vi "auto_id_subv.vi"(8 "error in":errorcluster, 9 "Amplitude":dbl=0.15 format="%#_13g", 10 "Bode amplitude 2":refnum<vi>, 11 "Swept-Sines-Control-Settings":cluster{"u-max":sgl, "offset":sgl, "Ki":sgl}) -> (0 "error out":errorcluster, 1 "Is-Totally-Stable":bool, 2 "Dinv-den":dbl[](array[numeric]) format="%#_10g", 3 "Dinv-num":dbl[](array[numeric]) format="%#_10g", 4 "fit_sos_result":T4)   [LabVIEW 2017]
uses:
  controls/SS_SweptSines.ctl
  controls/SS_sin_params.ctl
  controls/SS_input_data_json.ctl
  controls/fit_sos_results.ctl
  controls/SS_figures.ctl
  controls/bode_figure.ctl
  controls/SOS_frf_data.ctl
  controls/logging_selection.ctl
  <vilib>/Utility/error.llb/DialogType.ctl
  <vilib>/FPGAPlugInAG/cRIO-9082/niLvFpga_Open_cRIO-9082.vi
  <vilib>/rvi/interface/common/dynamic/niFpgaDynamicAddResources.vi
  <vilib>/FPGAPlugInAG/Dynamic/niLvFpga_Reset_Dynamic.vi
  <vilib>/rvi/interface/common/niFpgaWaitOnOcc.vi
  <vilib>/Utility/error.llb/Error Cluster From Error Code.vi
  <vilib>/rvi/errors/niLvFpgaAdjustHostInterfaceError.vi
  <vilib>/FPGAPlugInAG/Dynamic/niLvFpga_Run_Dynamic.vi
  <vilib>/FPGAPlugInAG/Dynamic/niLvFpga_Close_Dynamic.vi
  <vilib>/rvi/interface/nirviOpenFPGA/nirviOpenFPGA.xnode
  FPGA Bitfiles/SS_fpga_swept_sines.lvbitx
  <vilib>/rvi/interface/nirviMethod/nirviMethod.xnode
  <vilib>/rvi/interface/nirviReadWriteControl/nirviReadWriteControl.xnode
  <vilib>/rvi/interface/nirviCloseFPGA/nirviCloseFPGA.xnode
  NiFpgaLv.dll
  labview/utils_lib/utils.lvlib
  <vilib>/rvi/interface/Simulation/niFpgaSimulationCallBeginRW.vi
  <vilib>/FPGAPlugInAG/Dynamic/niLvFpga_ConfigureFifo_Dynamic.vi
  <vilib>/rvi/errors/niLvFpgaMergeErrorWithErrorCode.vi
panel:
  out "NaN/Path/Refnum?":bool
  in  "theta0":dbl[](array[numeric])=[0.6786, -1.9959, 0.99891, -1.996142, 0.9989]
  out "Freqs Done":i32(slide) scale=0.0..50.0
  out "SweptSines (out)":T1={"Log-Channel_select"=[FALSE, FALSE, FALSE, FALSE, FALSE, FALSE], "JSON Header"="", "SS-Params-Array"=[], "input_frequency_definitions"={"Amp"=0.0, "Ts"=0.0, "num_periodsMT"=[], "freqs_Hz"=[], "numAve_s"=[], "Nsamp_total"=[], "Nsettle_s"=[], "Ncollect_s"=[]}, "DAC-ADC primary 2"=0, "Channel-Names"=[], "num_chan"=0, "num-freqs"=0, "Input File (json)"=path "Z:/mpc-journal/sysID/FRF_data/x-axis_sines_info.json"} {"DAC-ADC primary 2" items=["DAC0/ADC0", "DAC1/ADC1", "DAC2/ADC2", "DAC3/ADC3", ""]}
  in  "Input File (json)":path=path "Z:/afm-cs/sysID/z-axis_sines_info_quick_firstRes.json"
  out "theta-fit":dbl[](array[numeric])
  out "Bode amplitude":cluster{"W":dbl[], "Magnitude":dbl[]}[](graph) caption="Magnitude Graph"
  in  "SweptSines (in)":T1={"Log-Channel_select"=[FALSE, FALSE, FALSE, FALSE, FALSE, FALSE], "JSON Header"="", "SS-Params-Array"=[], "input_frequency_definitions"={"Amp"=0.0, "Ts"=0.0, "num_periodsMT"=[], "freqs_Hz"=[], "numAve_s"=[], "Nsamp_total"=[], "Nsettle_s"=[], "Ncollect_s"=[]}, "DAC-ADC primary 2"=0, "Channel-Names"=[], "num_chan"=0, "num-freqs"=0, "Input File (json)"=path "Z:/afm-cs/sysID/x-axis_sines_info_intsamps_quick.json"} {"DAC-ADC primary 2" items=["DAC0/ADC0", "DAC1/ADC1", "DAC2/ADC2", "DAC3/ADC3", ""]}
  out "TsTicks":u32
  out "freq_adjusted":dbl
  in  "ABORT":bool
  out "boolean  indicators":T5
  out "number_of_freqs":i32
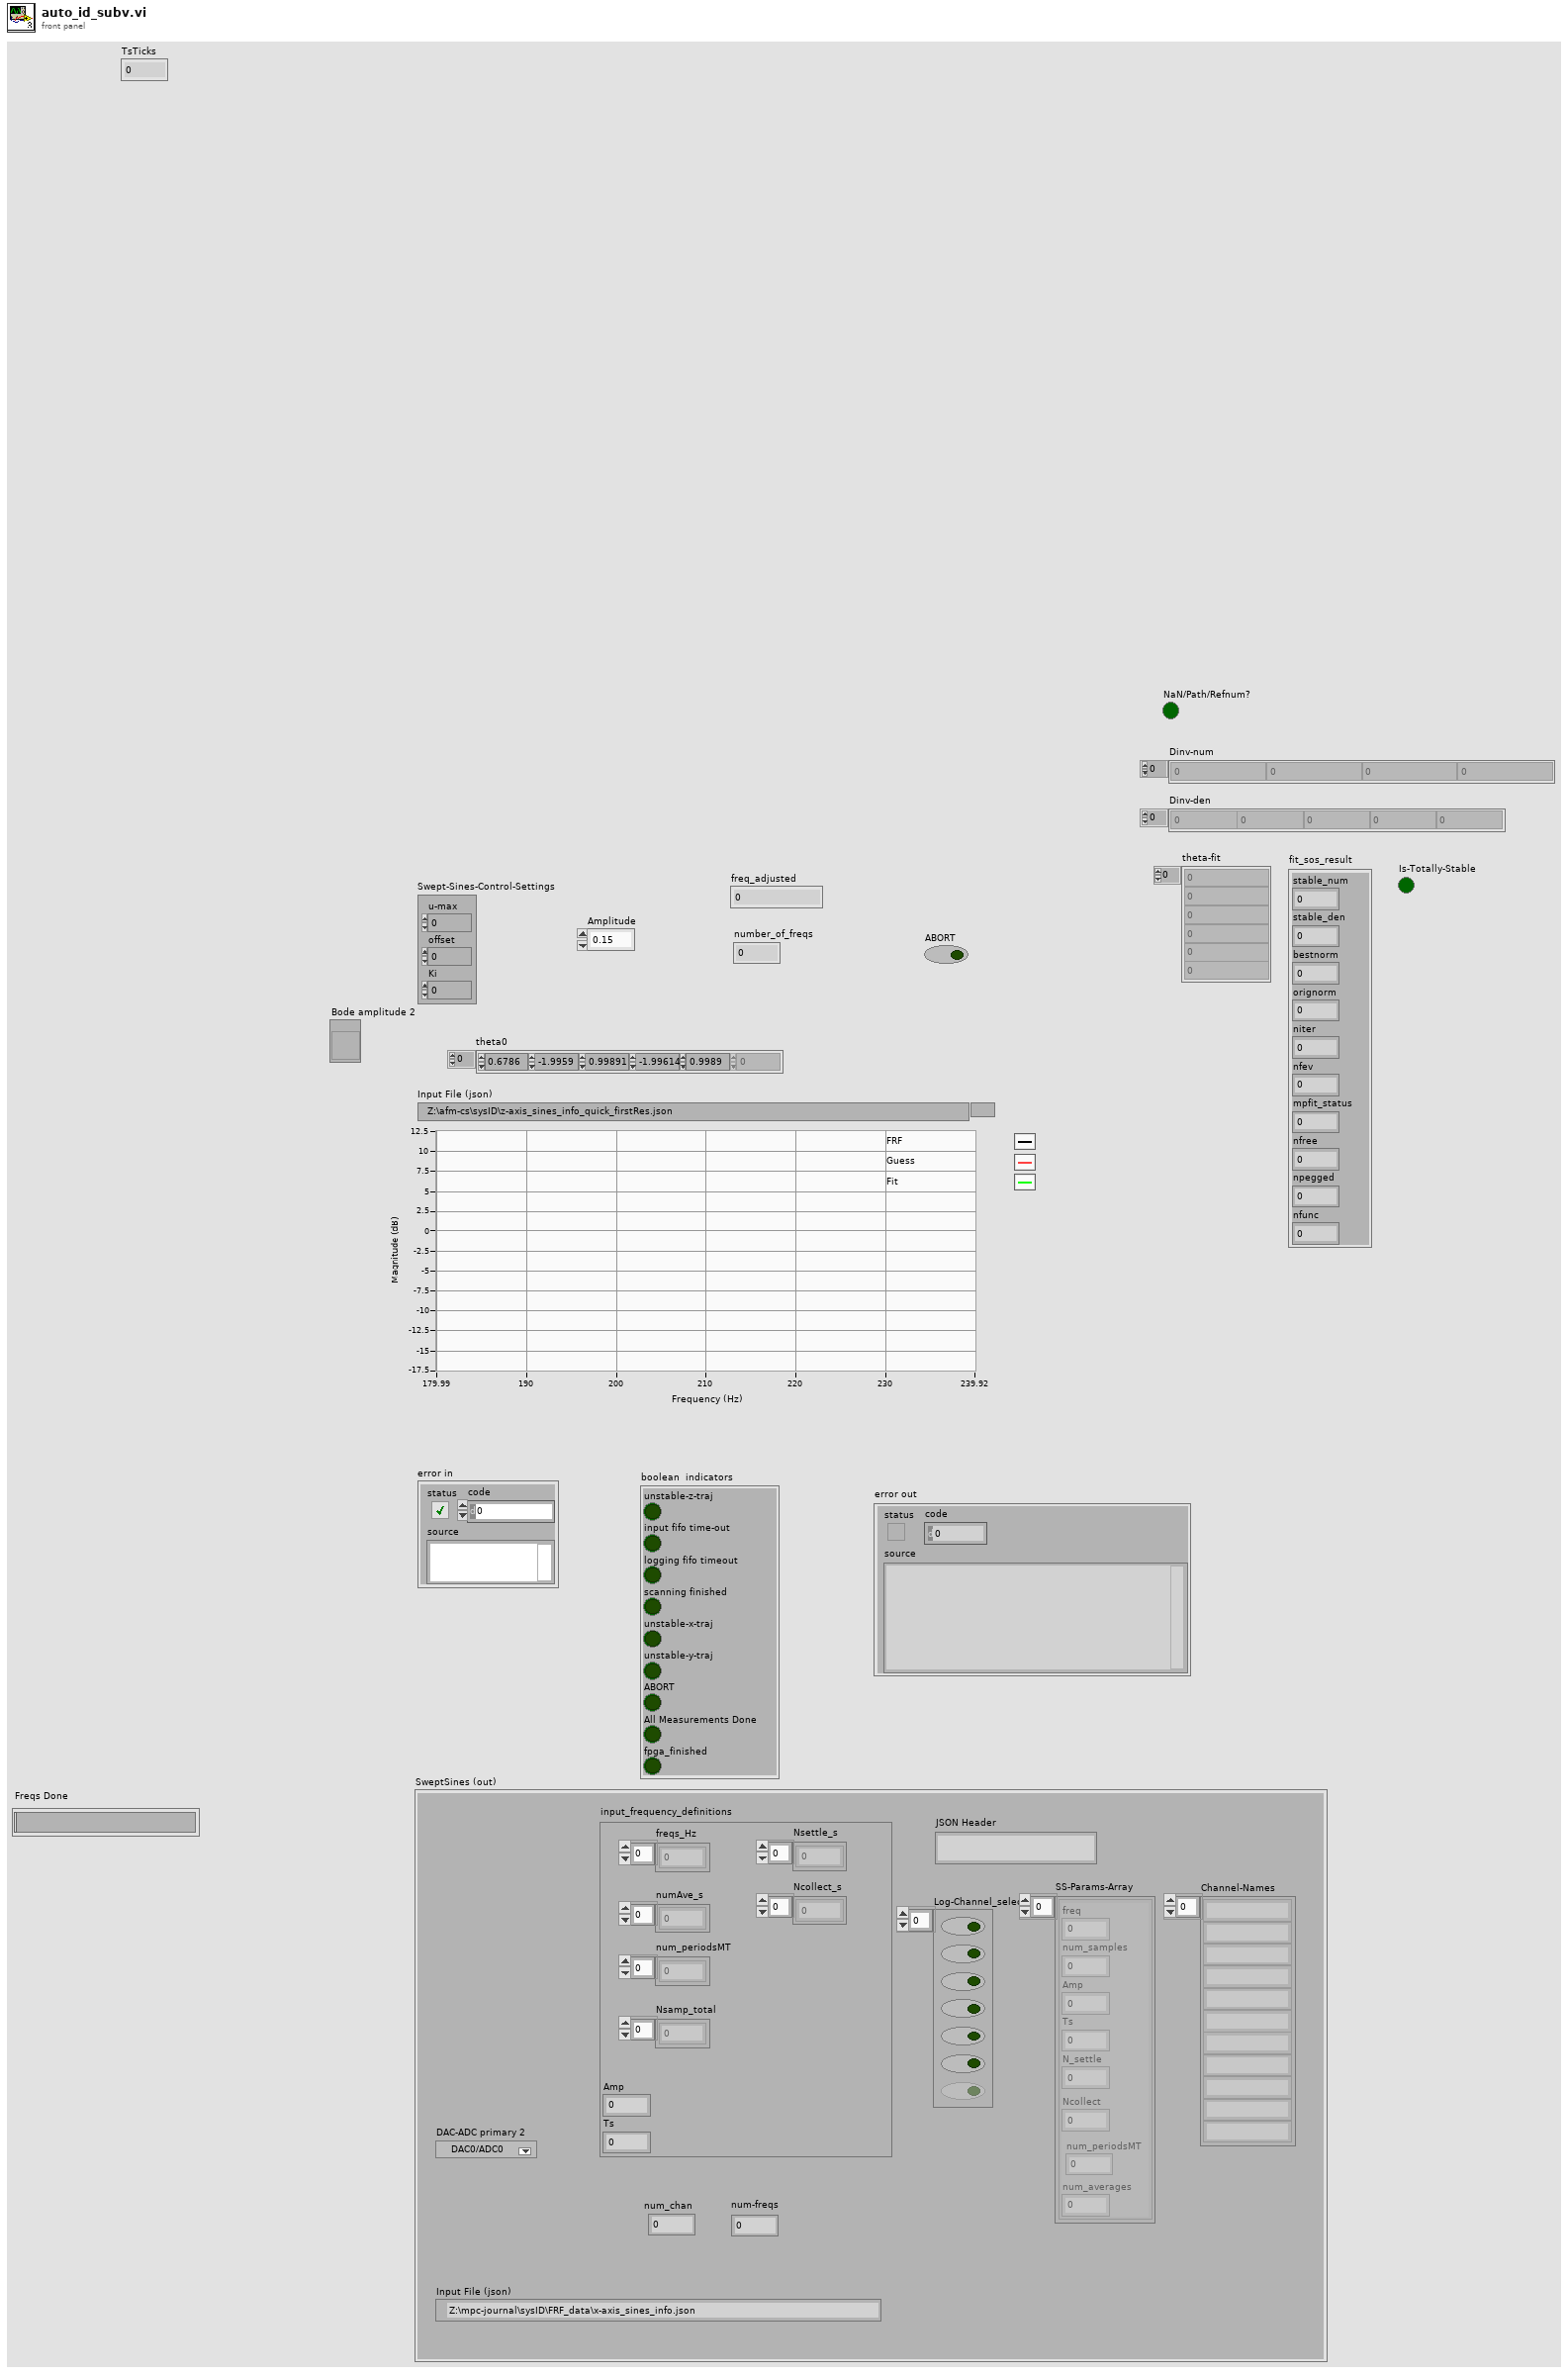
[diagram p1: front panel]
types:
  T1 = typedef "SS_SweptSines.ctl" = cluster{"Log-Channel_select":bool[], "JSON Header":string, "SS-Params-Array":T2[], "input_frequency_definitions":T3, "DAC-ADC primary 2":i16, "Channel-Names":string[], "num_chan":i32, "num-freqs":i32, "Input File (json)":path}
  T2 = typedef "SS_sin_params.ctl" = cluster{"freq":dbl, "num_samples":i32, "Amp":dbl, "Ts":dbl, "N_settle":u32, "Ncollect":i32, "num_periodsMT":i32, "num_averages":i32}
  T3 = typedef "SS_input_data_json.ctl" = cluster{"Amp":dbl, "Ts":dbl, "num_periodsMT":u32[], "freqs_Hz":dbl[], "numAve_s":i32[], "Nsamp_total":u32[], "Nsettle_s":u32[], "Ncollect_s":u32[]}
  T4 = typedef "fit_sos_results.ctl" = cluster{"stable_num":i32, "stable_den":i32, "bestnorm":dbl, "orignorm":dbl, "niter":i32, "nfev":i32, "mpfit_status":i32, "nfree":i32, "npegged":i32, "nfunc":i32}
  T5 = cluster{"unstable-z-traj":bool, "input fifo time-out":bool, "logging fifo timeout":bool, "scanning finished":bool, "unstable-x-traj":bool, "unstable-y-traj":bool, "ABORT":bool, "All Measurements Done":bool, "fpga_finished":bool}
  T6 = typedef "logging_selection.ctl" = cluster{"Collect reference":bool, "Collect DAC control":bool, "Collect AI-0":bool, "Collect AI-1":bool, "Collect AI-2":bool, "Collect AI-3":bool}
  T7 = typedef "SOS_frf_data.ctl" = cluster{"omegas":dbl[], "resp_real":dbl[], "resp_imag":dbl[], "theta0":dbl[]}
  T8 = typedef "SS_figures.ctl" = cluster{"bode figures":T9, "Freqs Done":refnum<vi>}
  T9 = typedef "bode_figure.ctl" = cluster{"Bode phase":refnum<vi>, "Bode amplitude":refnum<vi>}
  T10 = typedef "FrdData.ctl" = cluster{"Frequency Unit":enum16{"Hz", "rad/s"}, "W":dbl[], "MagDB":dbl[], "PhaseDeg":dbl[], "Resp":cdb[], "Data-name":string}
  T11 = typedef "DialogType.ctl" = u16
  T12 = typedef "SS_experimental-data.ctl" = cluster{"sin-data-out":dbl[][], "Fourier Data":T13, "freq_adjusted?":dbl, "below-nyquist":bool}
  T13 = typedef "SS_FourierData.ctl" = cluster{"E_s":dbl[], "Fourier Coefs":cdb[], "freq-adjusted":dbl}
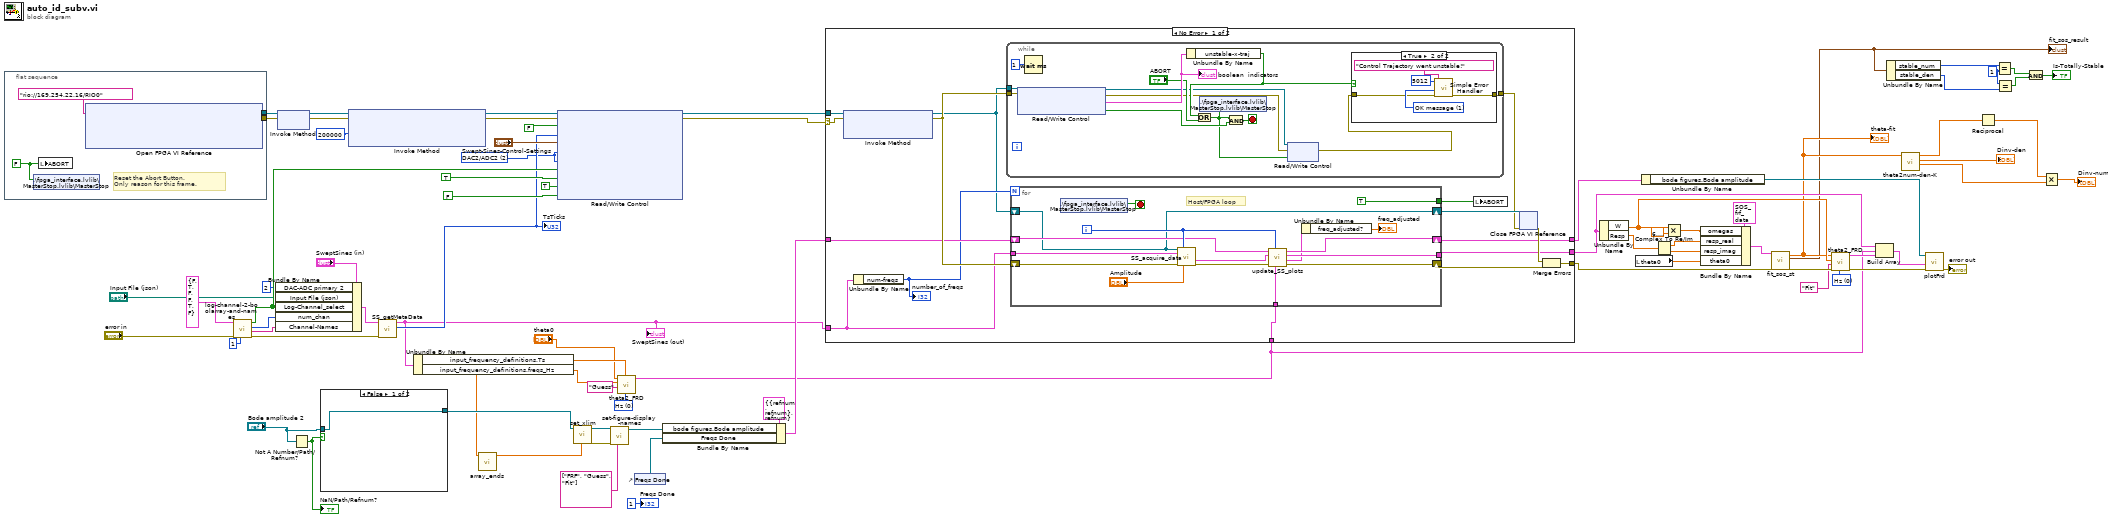
[diagram p0: block diagram]
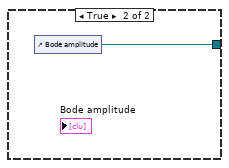
[diagram p2: hidden frame]
diagram:
  w7 = 1
  w55 = i16 2 items=["DAC0/ADC0", "DAC1/ADC1", "DAC2/ADC2", "DAC3/ADC3", ""] ("DAC-ADC primary")
  w39 = u16 0 items=["Hz", "rad/s"] ("freq unit")
  w48 = u16 0 items=["Hz", "rad/s"] ("freq unit")
  n1 = flat-sequence {
    tunnel: [w82] -> w78
    tunnel: [w81] -> w77
    frame #0 {
      w80 = FALSE
      # "Reset the Abort Button.\nOnly reason for this frame."
      n2 = shared-variable ".\\fpga_interface.lvlib\\MasterStop.lvlib\\MasterStop"(w80) -> ()  [unwired: 1 in, 1 out]
      n3 = local write "ABORT"(w80) -> ()
      n4 = xnode "Open FPGA VI Reference"("resource name"=tag "rio://169.254.22.16/RIO0") -> ("FPGA VI Reference Out"=w82:refnum<k20>, "error out"=w81:errorcluster)  [unwired: 1 in]
    }
  }
  n5 = call "log-channel-2-boolarray-and-names.vi"("min_number_chan"=i16 1, "error in"="error in", "Logging selection"=T6 {"Collect reference"=FALSE, "Collect DAC control"=TRUE, "Collect AI-0"=FALSE, "Collect AI-1"=FALSE, "Collect AI-2"=TRUE, "Collect AI-3"=FALSE}) -> ("error out"=w66:errorcluster, "Channel-Names"=w64:string[], "num_chan"=w61:i32, "Log-Channel_select"=w59:bool[])  [unwired: 5 in]
  n6 = Bundle By Name(cluster="SweptSines (in)", "DAC-ADC primary 2"=i16 2, "Input File (json)"="Input File (json)", "Log-Channel_select"=w59, "num_chan"=w61, "Channel-Names"=w64) -> (w63:T1)
  n7 = xnode "Invoke Method"("FPGA VI Reference In"=w78, "error in"=w77) -> ("FPGA VI Reference Out"=w71:refnum<k20>, "error out"=w70:errorcluster)
  n8 = Not A Number/Path/Refnum?(number/path/refnum="Bode amplitude 2") -> (NaN/Path/Refnum?=w2:bool)
  "NaN/Path/Refnum?" <- w2
  n9 = case shown="False" w2 {
    tunnel: [w84 w85] -> w53
    tunnel: "Bode amplitude 2" -> [w84 _]
    frame False {
    }
    frame True {
      n10 = control-ref of="Bode amplitude"() -> (w85:refnum<vi>)
    }
  }
  n11 = xnode "Invoke Method"("FPGA VI Reference In"=w71, "error in"=w70, "Requested Depth"=200000 ("requested depth")) -> ("FPGA VI Reference Out"=w76:refnum<k20>, "error out"=w72:errorcluster)  [unwired: 1 out]
  n12 = call "SS_getMetaData.vi"("error in"=w66, "SweptSines"=w63) -> ("TsTicks"=w56:u32, "SweptSines (out)"=w23:T1)  [unwired: 6 in, 1 out]
  "TsTicks" <- w56
  "SweptSines (out)" <- w23
  n13 = Unbundle By Name(w23) -> ("input_frequency_definitions.Ts"=w47:dbl, "input_frequency_definitions.freqs_Hz"=w46:dbl[])
  n14 = call "array_ends.vi"("freqs_Hz"=w46) -> ("Array"=w50:dbl[])  [unwired: 10 in]
  n15 = xnode "Read/Write Control"("FPGA VI Reference In"=w76, "error in"=w72, "ABORT"=FALSE, "TsTicks"=w56, "Swept-Sines-Control-Settings"="Swept-Sines-Control-Settings", "ADC-select"=w55, "DAC-select"=w55, "Log-Channel_select"=w59, "Subtract y0?"=TRUE ("Subtract-origin"), "reset"=TRUE, "Close Loop?"=FALSE) -> ("FPGA VI Reference Out"=w68:refnum<k20>, "error out"=w67:errorcluster)
  n16 = call "set_xlim.vi"("xlim"=w50, "figure (in)"=w53) -> ("error out"=w51:errorcluster, "figure (out)"=w52:refnum<vi>)  [unwired: 8 in]
  n17 = call "set-figure-display-names.vi"("DisplayNames"=string[] ["FRF", "Guess", "Fit"] ("Data_names"), "error in"=w51, "figure (in)"=w52) -> ("figure (out)"=w44:refnum<vi>)  [unwired: 7 in, 1 out]
  n18 = call "theta2_FRD.vi"("freq unit"=w48, "Sampling Time (s)"=w47, "Data-name"="Guess", "freqs/omega"=w46, "theta"="theta0") -> ("FRD-model"=w24:T10)  [unwired: 5 in, 1 out]
  n19 = control-ref of="Freqs Done"() -> (w18:refnum<vi>)
  n20 = Bundle By Name(cluster=T8 {"bode figures"={"Bode phase"=refnum, "Bode amplitude"=refnum}, "Freqs Done"=refnum} ("figures"), "bode figures.Bode amplitude"=w44, "Freqs Done"=w18) -> (w43:T8)
  n21 = case shown="No Error" w67 {
    selector: w67 -> [w91 w138]
    tunnel: w68 -> [w101 _]
    tunnel: [w96 w138] -> w54
    tunnel: w23 -> [w93 _]
    tunnel: w43 -> [w94 w137]
    tunnel: [w89 w137] -> w30
    tunnel: w24 -> [w88 _]
    tunnel: [w87 _] -> w25
    frame No Error {
      n22 = xnode "Invoke Method"("FPGA VI Reference In"=w101, "error in"=w91) -> ("FPGA VI Reference Out"=w86:refnum<k20>, "error out"=w99:errorcluster)  [unwired: 1 in]
      n23 = Unbundle By Name(w93) -> ("num-freqs"=w92:i32)
      "number_of_freqs" <- w92
      n24 = while {
        tunnel: w86 -> [w113]
        tunnel: w99 -> [w112]
        tunnel: [w108] -> w95
        stop <- w104 stop-if-true
        n25 = xnode "Read/Write Control"("FPGA VI Reference In"=w113, "error in"=w112) -> ("FPGA VI Reference Out"=w107:refnum<k20>, "error out"=w106:errorcluster, "boolean  indicators"=w111:T5, "All Done"=w103:bool)
        "boolean  indicators" <- w111
        n26 = Wait (ms)(milliseconds to wait=u32 1) -> ()  [unwired: 1 out]
        n27 = Unbundle By Name(w111) -> ("unstable-x-traj"=w109:bool)
        n28 = Or(x=w109, y="ABORT") -> (x .or. y?=w102:bool)
        n29 = shared-variable ".\\fpga_interface.lvlib\\MasterStop.lvlib\\MasterStop"(w102) -> ()  [unwired: 1 in, 1 out]
        n30 = And(x=w102, y=w103) -> (x .and. y?=w104:bool)
        n31 = xnode "Read/Write Control"("FPGA VI Reference In"=w107, "error in"=w106, "ABORT"=w102) -> ("error out"=w105:errorcluster)  [unwired: 1 out]
        n32 = case shown="True" w109 {
          tunnel: w105 -> [w115 w117]
          tunnel: [w115 w116] -> w108
          frame False {
          }
          frame True {
            w120 = T11 1 items=["no dialog", "OK message", "continue or stop message", "OK message + warnings", "continue/stop + warnings"] ("type of dialog (OK msg:1)")
            n33 = call <vilib>:"Simple Error Handler.vi"("error code (no error:0)"=5012, "error source (\" \")"="Control Trajectory went unstable!" ("error source (\" \")"), "type of dialog (OK msg:1)"=w120, "error in (no error)"=w117) -> ("error out"=w116:errorcluster)  [unwired: 1 in, 4 out]
          }
        }
      }
      n34 = for {
        N: w92 -> [_]
        shift-right: [w126] -> w89
        shift-left: w94 -> [w125]
        tunnel: [TRUE] -> w98
        shift-right: [w132] -> w90
        shift-left: w99 -> [w134]
        tunnel: w93 -> [w133]
        tunnel: [w127] -> w87
        tunnel: w88 -> [w123]
        shift-right: [w121] -> w100
        shift-left: w86 -> [w121]
        i -> [w130]
        stop <- w122 stop-if-true
        # "Host/FPGA loop"
        n35 = shared-variable ".\\fpga_interface.lvlib\\MasterStop.lvlib\\MasterStop"() -> (w122:bool)  [unwired: 1 in, 1 out]
        n36 = call "SS_acquire_data.vi"("Type"=w121, "idx"=w130, "SweptSines (in)"=w133, "error in"=w134, "Signal Amplitude (V)"="Amplitude") -> ("experiment-data"=w129:T12, "error IO"=w128:errorcluster)  [unwired: 7 in, 2 out]
        n37 = call "update_SS_plots.vi"("other-frd"=w123, "freqs-iter"=w130, "error in (no error)"=w128, "experiment-data"=w129, "figures-in"=w125) -> ("error out"=w132:errorcluster, "experiment-data (out)"=w124:T12, "FRD-out"=w127:T10, "figures-out"=w126:T8)  [unwired: 3 in]
        n38 = Unbundle By Name(w124) -> ("freq_adjusted?"=→"freq_adjusted":dbl)
      }
      n39 = local write "ABORT"(w98) -> ()
      n40 = xnode "Close FPGA VI Reference"("FPGA VI Reference In"=w100, "error in"=w95) -> ("error out"=w97:errorcluster)
      n41 = Merge Errors(w97, w90) -> (w96:errorcluster)
    }
    frame Error {
    }
  }
  n42 = Unbundle By Name(w25) -> ("W"=w17:dbl[], "Resp"=w32:cdb[])
  n43 = local read "theta0"() -> (w31:dbl[])
  n44 = Unbundle By Name(w30) -> ("bode figures.Bode amplitude"=w26:refnum<vi>)
  n45 = Complex To Re/Im(x + iy=w32) -> (x=w34:dbl[], y=w33:dbl[])
  n46 = Multiply(x=w17, y=6.283185307179586) -> (x*y=w36:dbl[])
  n47 = Bundle By Name(cluster=T7 {"omegas"=[1006.674891, 1016.262272, 1025.849652, 1035.437033, 1045.024413, 1054.611794, 1064.199174, 1073.786548, 1083.373929, 1092.961309, 1102.54869, 1112.13607, 1121.723451, 1131.310831, 1140.898212, 1150.485592, 1160.072973, 1169.660354, 1179.247728, 1188.835108, 1198.422489, 1208.009869, 1217.59725, 1227.18463, 1236.772011, 1246.359391, 1255.946772, 1265.534152, 1275.121533, 1284.708907, 1294.296288, 1303.883668, 1313.471049, 1323.058429, 1332.64581, 1342.23319, 1351.820571, 1361.407951, 1370.995332, 1380.582706, 1390.170086, 1399.757467, 1409.344847, 1418.932228, 1428.519609, 1438.106989, 1447.69437, 1457.28175, 1466.869131, 1476.456511, 1486.043885, 1495.631266, 1505.218646, 1514.806027, 1524.393407, 1533.980788, 1543.568168, 1553.155549, 1562.742929, 1572.33031, 1581.91769, 1591.505065, 1601.092445, 1610.679826, 1620.267206, 1629.854587, 1639.441967, 1649.029348, 1658.616728], "resp_real"=[0.6710936201, 0.6732167298, 0.6736550301, 0.6739624194, 0.6764113406, 0.6760996891, 0.6752809587, 0.67695858, 0.6764911126, 0.6818501379, 0.6804259731, 0.6777421689, 0.683602427, 0.6839502494, 0.6873055899, 0.6871681129, 0.6836241729, 0.6933718335, 0.6965190689, 0.7011525702, 0.7041006273, 0.7087951209, 0.7138881005, 0.7230810664, 0.7347158563, 0.743593779, 0.7581554602, 0.7740064901, 0.7983882262, 0.8168799192, 0.8500537495, 0.885993569, 0.8534751304, 0.6135298299, 0.1963078728, 0.06997493602, 0.2143720387, 0.3262401307, 0.3874363268, 0.4244315327, 0.4518076771, 0.4783094111, 0.4942330365, 0.5078067569, 0.5183774173, 0.5254372068, 0.5346584888, 0.5422376, 0.5476692529, 0.546204086, 0.5501300272, 0.5526801006, 0.557631838, 0.5639162136, 0.5601299408, 0.5627301292, 0.5646599194, 0.5678509651, 0.5674161925, 0.5676099823, 0.5703128211, 0.5717199117, 0.5717616028, 0.5714305364, 0.5706488864, 0.574491682, 0.5720673373, 0.5722619255, 0.5727540208], "resp_imag"=[0.1828230252, 0.185702312, 0.1893108783, 0.1927179342, 0.1939516982, 0.1991804891, 0.1996588255, 0.1997489381, 0.2009184192, 0.2058333084, 0.205968755, 0.2071290225, 0.2120033665, 0.2140896781, 0.2197333799, 0.2218060221, 0.2270970718, 0.2243543787, 0.2282290931, 0.2349554807, 0.2362899955, 0.2386023634, 0.2479762836, 0.2514213949, 0.2589829258, 0.2690734156, 0.2817668466, 0.3075000844, 0.3292949756, 0.3581777586, 0.418098085, 0.518537997, 0.7274335428, 0.9954410219, 0.8283414758, 0.4651799029, 0.2632646215, 0.2204933474, 0.2100370796, 0.215817828, 0.2094899805, 0.2041701149, 0.2090161752, 0.2122336611, 0.2144513636, 0.2154505064, 0.2184072105, 0.2207006189, 0.2264320741, 0.2319746485, 0.2352243002, 0.2359211056, 0.2344839067, 0.234200787, 0.2350554818, 0.2419460399, 0.2451480379, 0.2422561944, 0.2450402058, 0.2520603413, 0.2526693987, 0.2530329194, 0.2523935129, 0.2570623818, 0.2576871444, 0.2563998974, 0.259830217, 0.2610581842, 0.2647075477], "theta0"=[0.6786, -1.9959, 0.99891, -1.996142, 0.9989]} ("SOS-frf_data"), "omegas"=w36, "resp_real"=w34, "resp_imag"=w33, "theta0"=w31) -> (w37:T7)
  n48 = call "fit_sos_st.vi"("frf_data"=w37, "error in (no error)"=w54) -> ("theta"=w16:dbl[], "fit_sos_result"=w10:T4, "error out"=w41:errorcluster)  [unwired: 23 in]
  "fit_sos_result" <- w10
  "theta-fit" <- w16
  n49 = call "theta2_FRD.vi"("freq unit"=w39, "error in (no error)"=w41, "Data-name"="Fit", "freqs/omega"=w17, "theta"=w16) -> ("error out"=w27:errorcluster, "FRD-model"=w29:T10)  [unwired: 5 in]
  n50 = Build Array(w25, w24, w29) -> (w28:T10[])
  n51 = Unbundle By Name(w10) -> ("stable_num"=w9:i32, "stable_den"=w8:i32)
  n52 = call "theta2num-den-K.vi"("theta"=w16) -> ("Den"=w13:dbl[], "Num"=→"Dinv-den":dbl[], "K"=w14:dbl)  [unwired: 8 in]
  n53 = call "plotFrd.vi"("error in (no error)"=w27, "FRD-array"=w28, "Magnitude Graph Reference in"=w26) -> ("error out"=→"error out":errorcluster)  [unwired: 6 in, 2 out]
  n54 = Reciprocal(x=w14) -> (1/x=w11:dbl)
  n55 = Equal?(x=w9, y=w7) -> (x = y?=w5:bool)
  n56 = Equal?(x=w7, y=w8) -> (x = y?=w6:bool)
  n57 = And(x=w5, y=w6) -> (x .and. y?=→"Is-Totally-Stable":bool)
  n58 = Multiply(x=w11, y=w13) -> (x*y=→"Dinv-num":dbl[])
  "Freqs Done" <- 1 ("Freqs Done")
